vi "Generate Array (SubVI).vi"(8 "error in (no error)":errorcluster, 9 "Final":dbl=5.4 format="%_6g", 10 "Step":dbl=0.1 format="%_6g", 11 "Initial":dbl=0.7 format="%_6g") -> (0 "error out":errorcluster, 2 "Array size":i32, 3 "Array out":dbl[](array[numeric])=[0.7, 0.7999999999999999, 0.8999999999999999, 1.0, 1.1, 1.2, 1.3, 1.4, 1.5, 1.6, 1.7, 1.8, 1.9000000000000001, 2.0, 2.1, 2.2, 2.3, 2.4000000000000004, 2.5, 2.6, 2.7, 2.8, 2.9000000000000004, 3.0, 3.1000000000000005, 3.2, 3.3, 3.4000000000000004, 3.5, 3.6000000000000005, 3.7, 3.8, 3.9000000000000004, 4.0, 4.1000000000000005, 4.2, 4.3, 4.4, 4.5, 4.6000000000000005, 4.7, 4.800000000000001, 4.9, 5.0, 5.1000000000000005, 5.2, 5.300000000000001])   [LabVIEW 2020]
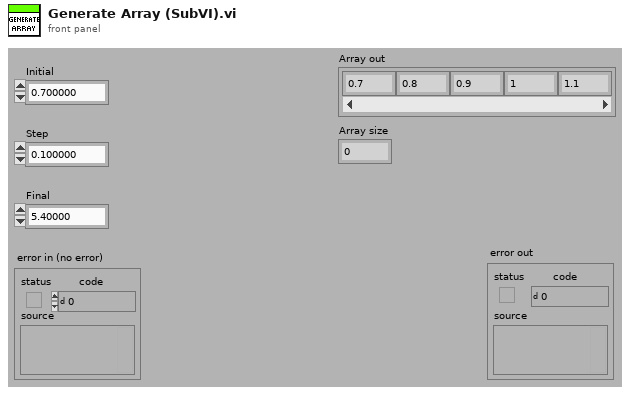
[diagram p1: front panel]
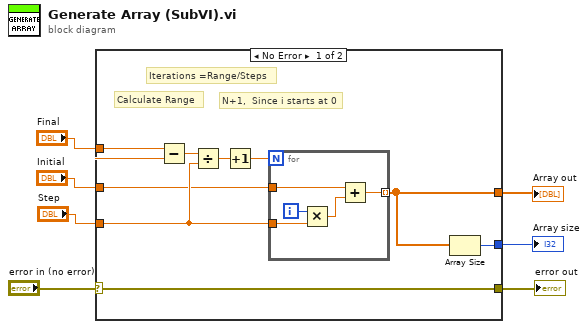
[diagram p0: block diagram]
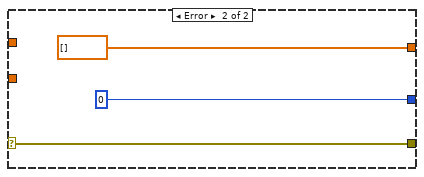
[diagram p2: hidden frame]
diagram:
  n1 = case shown="No Error" "error in (no error)" {
    selector: "error in (no error)" -> [w8 w24]
    tunnel: [w8 w24] -> w6
    tunnel: "Step" -> [w13 _]
    tunnel: "Final" -> [w12 _]
    tunnel: "Initial" -> [w11 _]
    tunnel: [w10 dbl[] []] -> w2
    tunnel: [w9 0] -> w1
    frame No Error {
      # "N+1,  Since i starts at 0"
      # "Iterations =Range/Steps"
      # "Calculate Range"
      n2 = Subtract ("Range")(x=w12, y=w11) -> (x-y=w14:dbl)
      n3 = Divide(x=w14, y=w13) -> (x/y=w15:dbl)
      n4 = Increment(x=w15) -> (x+1=w16:dbl)
      n5 = for {
        N: w16 -> [_]
        tunnel: w13 -> [w20]
        tunnel: w11 -> [w19]
        tunnel: [w17] -> w10 mode=indexing
        i -> [w21]
        n6 = Multiply(x=w21, y=w20) -> (x*y=w18:dbl)
        n7 = Add(x=w19, y=w18) -> (x+y=w17:dbl)
      }
      n8 = Array Size(array=w10) -> (size(s)=w9:i32)
    }
    frame Error {
    }
  }
  "error out" <- w6
  "Array out" <- w2
  "Array size" <- w1
